vi "To Serial Form.vi"(8 "error in (no error)":errorcluster, 9 "Metadata":variant, 10 "CI Serializer in":refnum<class "CI Serializer.lvclass">, 11 "CI Project in":refnum<class "CI Project.lvclass">) -> (0 "error out":errorcluster, 1 "Serialized Job Name":string, 2 "CI Serializer out":refnum<class "CI Serializer.lvclass">, 3 "CI Project out":refnum<class "CI Project.lvclass">)   [LabVIEW 2014, in "CI Project.lvclass"]
uses:
  CI Project.lvclass
  CI Serializer/CI Serializer.lvclass
  <vilib>/ni/Configuration Framework/Node/NISE_CEF_Node.lvclass/NISE_CEF_Node.ctl
  Serializable Node/Serializable Node.lvclass
  <vilib>/ni/Configuration Framework/Node/ReadChildren.vi
  Build Job/Build Job.lvclass
  <vilib>/ni/Configuration Framework/Node/NISE_CEF_Node.lvclass
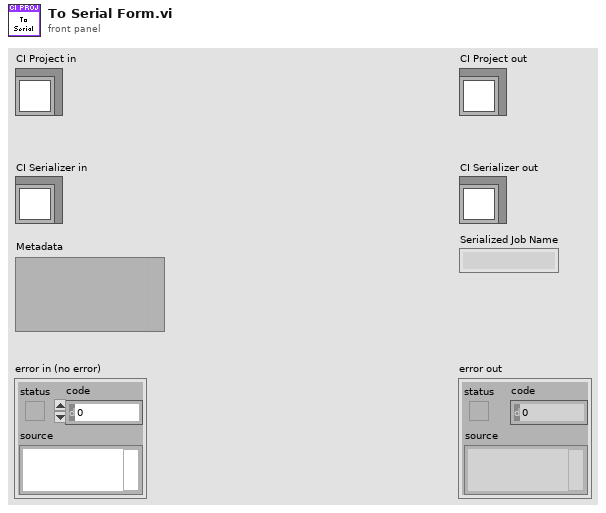
[diagram p1: front panel]
types:
  T1 = typedef "NISE_CEF_Node.lvclass/NodeRef.ctl" = refnum<data-value>
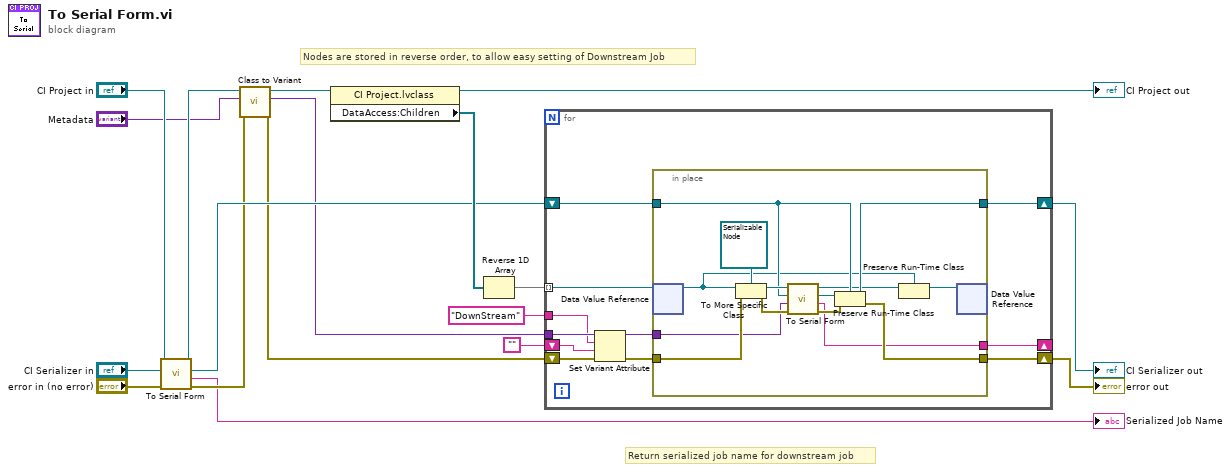
[diagram p0: block diagram]
diagram:
  # "Return serialized job name for downstream job"
  # "Nodes are stored in reverse order, to allow easy setting of Downstream Job"
  n1 = call-parent "To Serial Form.vi"("error in (no error)"="error in (no error)", "CI Serializer in"="CI Serializer in", "Serializable Node in"="CI Project in") -> ("error out"=w11:errorcluster, "Serialized Job Name"=→"Serialized Job Name":string, "CI Serializer out"=w16:refnum<class "CI Serializer.lvclass">, "Serializable Node out"=w8:refnum<class "CI Project.lvclass">)  [unwired: 5 in]
  n2 = call-dynamic "Class to Variant.vi"("error in (no error)"=w11, "Data in"="Metadata", "CI Project in"=w8) -> ("error out"=w10:errorcluster, "Data Out"=w12:variant, "CI Project out"=w13:refnum<class "CI Project.lvclass">)  [unwired: 5 in, 1 out]
  n3 = property class="CI Project.lvclass"(reference=w13) -> (reference out=→"CI Project out":refnum<class "CI Project.lvclass">, "DataAccess:Children"=w17:T1[])  [unwired: 1 in, 1 out]
  n4 = Reverse 1D Array(array=w17) -> (reversed array=w7:T1[])
  n5 = for {
    tunnel: w7 -> [w21] mode=indexing
    tunnel: w12 -> [w28]
    shift-right: [w22] -> w4
    shift-left: w16 -> [w23]
    shift-right: [w20] -> w3
    shift-left: w10 -> [w29]
    tunnel: "DownStream" ("name") -> [w27]
    shift-right: [w19] -> _
    shift-left: "" -> [w26]
    n6 = Set Variant Attribute(Variant=w28, name=w27, value=w26, error in=w29) -> (Variant out=w24:variant, error out=w25:errorcluster)  [unwired: 1 out]
    n7 = in-place {
      in-place-border: w23 -> [w38]
      in-place-border: [w37] -> w22
      in-place-border: w25 -> [w36]
      in-place-border: [w32] -> w20
      in-place-border: w24 -> [w31]
      in-place-border: [w30] -> w19
      n8 = in-place-dvr #1(w21) -> (w33:refnum<class "NISE_CEF_Node.lvclass">)  [unwired: 1 out]
      n9 = To More Specific Class(target class=refnum<class "Serializable Node.lvclass"> refnum ("Serializable Node in"), reference=w33, error in=w36) -> (specific class reference=w39:refnum<class "Serializable Node.lvclass">, error out=w41:errorcluster)
      n10 = call-dynamic "To Serial Form.vi"("error in (no error)"=w41, "Metadata"=w31, "CI Serializer in"=w38, "Serializable Node in"=w39) -> ("error out"=w43:errorcluster, "Serialized Job Name"=w30:string, "CI Serializer out"=w42:refnum<class "CI Serializer.lvclass">, "Serializable Node out"=w35:refnum<class "Serializable Node.lvclass">)  [unwired: 4 in]
      n11 = Preserve Run-Time Class(object in=w42, error in=w43, 2:w38) -> (object out=w37:refnum<class "CI Serializer.lvclass">, error out=w32:errorcluster)
      n12 = Preserve Run-Time Class(object in=w35, 2:w33) -> (object out=w34:refnum<class "NISE_CEF_Node.lvclass">)  [unwired: 1 in, 1 out]
      n13 = in-place-dvr #1(w34) -> ()  [unwired: 2 out]
    }
  }
  "error out" <- w3
  "CI Serializer out" <- w4
